vi "Nested Tests.vi"(8 "error in":errorcluster) -> (0 "error out":errorcluster)   [LabVIEW 2020, in "Caraya Extension Tests.lvclass"]
uses:
  Caraya Extension Tests.lvclass
  <vilib>/addons/_JKI Toolkits/Caraya/classes/Test/Test.lvclass
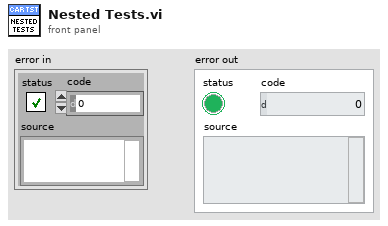
[diagram p1: front panel]
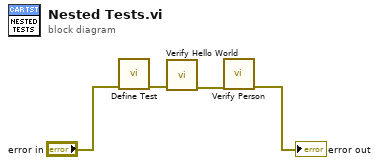
[diagram p0: block diagram]
diagram:
  n1 = call <vilib>:"Define Test.vi"("error in (no error)"="error in") -> ("error out"=w3:errorcluster)  [unwired: 9 in, 1 out]
  n2 = call "Verify Hello World.vi"("error in"=w3) -> ("error out"=w4:errorcluster)  [unwired: 10 in]
  n3 = call "Verify Person.vi"("error in"=w4) -> ("error out"=→"error out":errorcluster)  [unwired: 10 in]
